vi "Open Device.vi"() -> (0 "error out":errorcluster, 3 ".NET Refnum out":refnum<k24>)   [LabVIEW 2019, in "ESP301.lvlib"]
uses:
  ESP301.lvlib
  Newport.ESP301.CommandInterface
  <vilib>/Utility/config.llb/Read Key (String).vi
  <vilib>/Utility/config.llb/NI_LVConfig.lvlib
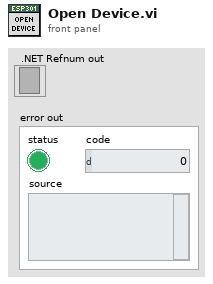
[diagram p1: front panel]
types:
  T1 = typedef "NI_LVConfig.lvlib/Config Data RefNum.ctl" = refnum<k1>
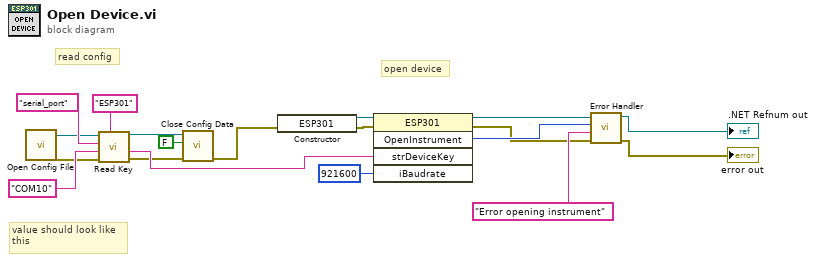
[diagram p0: block diagram]
diagram:
  # "read config"
  # "open device"
  # "value should look like\nthis"
  n1 = call "Open Config File.vi"() -> ("error out"=w5:errorcluster, "Refnum out"=w4:T1)  [unwired: 10 in]
  n2 = call-poly <vilib>:"Read Key.vi"("section"="ESP301", "error in (no error)"=w5, "default value"="COM10", "key"="serial_port", "refnum"=w4) -> ("error out"=w9:errorcluster, "value"=w18:string, "refnum out"=w10:T1)  [unwired: 3 in, 1 out]
  n3 = call <vilib>:"Close Config Data.vi"("error in (no error)"=w9, "write file if changed (T)"=FALSE, "refnum"=w10) -> ("error out"=w12:errorcluster)  [unwired: 7 in, 1 out]
  n4 = constructor class="ESP301"(error in=w12) -> (reference out=w2:refnum<k24>, error out=w1:errorcluster)  [unwired: 2 in, 1 out]
  n5 = invoke class="ESP301" method="OpenInstrument"(reference=w2, error in=w1, "strDeviceKey"=w18, "iBaudrate"=921600) -> (reference out=w15:refnum<k24>, error out=w13:errorcluster, "OpenInstrument"=w17:i32)  [unwired: 1 in, 2 out]
  n6 = call "Error Handler.vi"("error in (no error)"=w13, "value"="Error opening instrument", "OpenInstrument"=w17, ".NET Refnum in"=w15) -> ("error out"=→"error out":errorcluster, ".NET Refnum out"=→".NET Refnum out":refnum<k24>)  [unwired: 6 in]
